vi "CreateBusVirtualChannel.vi"(8 "error in (no error)":errorcluster, 10 "Wfm Data in":waveform(sgl)[](array[waveform]), 11 "Virtual Channel in":T1) -> (0 "error out":errorcluster, 1 "Created Bus Channel":waveform(sgl), 2 "Wfm Data out":waveform(sgl)[](array[waveform]), 3 "Virtual Channel out":T1)   [LabVIEW 2017, in "McsaVirtualChannel.lvlib"]
uses:
  <vilib>/addons/InsightCM/Devices/Shared/Mcsa/McsaVirtualChannel/McsaVirtualChannel.lvlib
  <vilib>/addons/InsightCM/Devices/Shared/Mcsa/McsaVirtualChannel/controls/VirtualChannel.ctl
  <vilib>/addons/InsightCM/Utilities/MCSA/McsaUtilities.lvlib
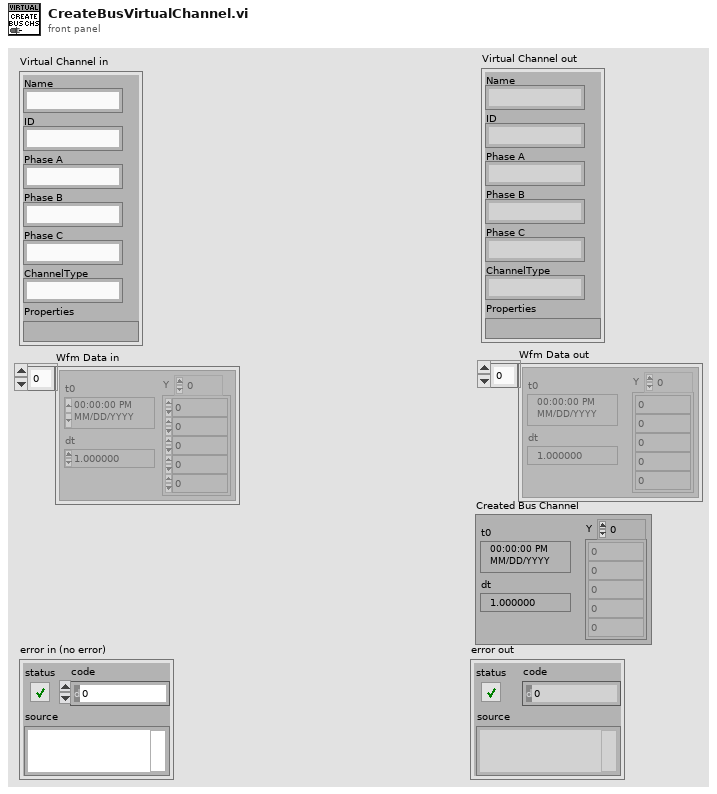
[diagram p1: front panel]
types:
  T1 = typedef "McsaVirtualChannel.lvlib/VirtualChannel.ctl" = cluster{"Name":string, "ID":string, "Phase A":string, "Phase B":string, "Phase C":string, "ChannelType":string, "Properties":variant}
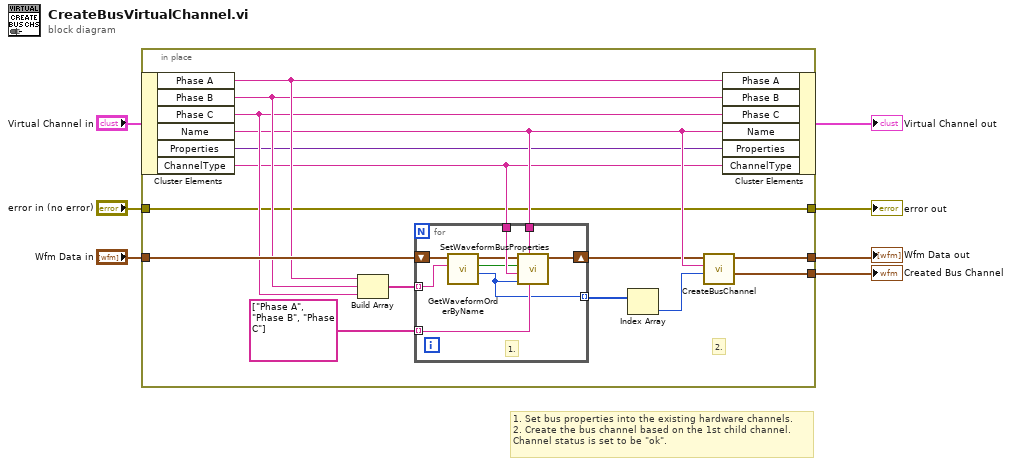
[diagram p0: block diagram]
diagram:
  # "1. Set bus properties into the existing hardware channels.\n2. Create the bus channel based on the 1st child channel.\nChannel status is set to be \"ok\"."
  n1 = in-place {
    in-place-border: "Wfm Data in" -> [w22]
    in-place-border: "error in (no error)" -> [w14]
    in-place-border: [w14] -> w3
    in-place-border: [w8] -> w2
    in-place-border: [w9] -> w1
    # "2."
    n2 = in-place-cluster #1("Virtual Channel in") -> ("Phase A"=w21:string, "Phase B"=w20:string, "Phase C"=w19:string, "Name"=w17:string, "Properties"=w13:variant, "ChannelType"=w16:string)
    n3 = Build Array(w21, w20, w19) -> (w18:string[])
    n4 = for {
      shift-right: [w31] -> w10
      shift-left: w22 -> [w27]
      tunnel: string[] ["Phase A", "Phase B", "Phase C"] -> [w29] mode=indexing
      tunnel: w18 -> [w26] mode=indexing
      tunnel: w17 -> [w30]
      tunnel: w16 -> [w28]
      tunnel: [w23] -> w12 mode=indexing
      # "1."
      n5 = call <vilib>:"GetWaveformOrderByName.vi"("Channel Name"=w26, "Acq Waveforms"=w27) -> ("Waveform Channel Order"=w23:i32, "Found?"=w24:bool, "Acq Waveforms Out"=w25:waveform(sgl)[])  [unwired: 6 in, 1 out]
      n6 = call <vilib>:"SetWaveformBusProperties.vi"("Phase Order"=w29, "Bus Channel Name"=w30, "Waveform Channel Order"=w23, "Channel Type"=w28, "Found?"=w24, "all channels Wfm"=w25) -> ("all channels Wfm"=w31:waveform(sgl)[])  [unwired: 5 in]
    }
    n7 = Index Array(array=w12) -> (element=w11:i32)  [unwired: 1 in]
    n8 = call <vilib>:"CreateBusChannel.vi"("1st child channel index"=w11, "Bus Name"=w17, "Wfm Data in"=w10) -> ("Created Bus Channel"=w8:waveform(sgl), "Wfm Data out"=w9:waveform(sgl)[])  [unwired: 7 in]
    n9 = in-place-cluster #1("Phase A"=w21, "Phase B"=w20, "Phase C"=w19, "Name"=w17, "Properties"=w13, "ChannelType"=w16) -> (→"Virtual Channel out":T1)
  }
  "error out" <- w3
  "Created Bus Channel" <- w2
  "Wfm Data out" <- w1
